vi "numberToAutoEnum.vi"(10 "inNumber":dbl) -> (2 "outEnum":T1(ring))   [LabVIEW 2017]
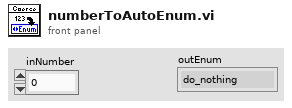
[diagram p1: front panel]
types:
  T1 = enum16{"do_nothing", "cross_baseline_short", "cross_baseline_long", "hot_from_middle", "if_hot_2_cube_else_1_cube", "if_hot_1_cube_else_1_cube", "exchange_from_middle", "forward_switch_if_hot", "exchange_from_outside", "if_hot_2_cube_else_baseline", "if_hot_3_cube_else_baseline", "exchange_and_hot_switch", "hot_from_middle_diagonal", "yet to be named", "If_hot_1_else_baseline", "hot_2_from_middle", "motion_profiling_test"}
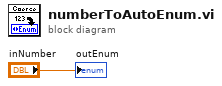
[diagram p0: block diagram]
diagram:
  "outEnum" <- "inNumber"
